vi "update settings and acquire.vi"(8 "error in (no error)":errorcluster, 10 "Settings In":T1, 11 "Queue in":refnum<queue>) -> (0 "error out":errorcluster)   [LabVIEW 2014, in "AvaSpec.lvlib"]
uses:
  AvaSpec.lvlib
  Message Queue/Message Cluster.ctl
  Settings/Settings.ctl
  Acquisition/Hardware Configuration.ctl
  Libraries/AS-5216-DLL/AVS settings.ctl
  Acquisition/Sphere Indicator.ctl
  Settings/Measurement Type.ctl
  Logging/Logging Configuration.ctl
  Message Queue/AvaSpec Message Queue.lvlib
  Acquisition/AvaSpec Acquisition.lvlib
  Logging/AvaSpec Logging.lvlib
  Settings/AvaSpec Settings.lvlib
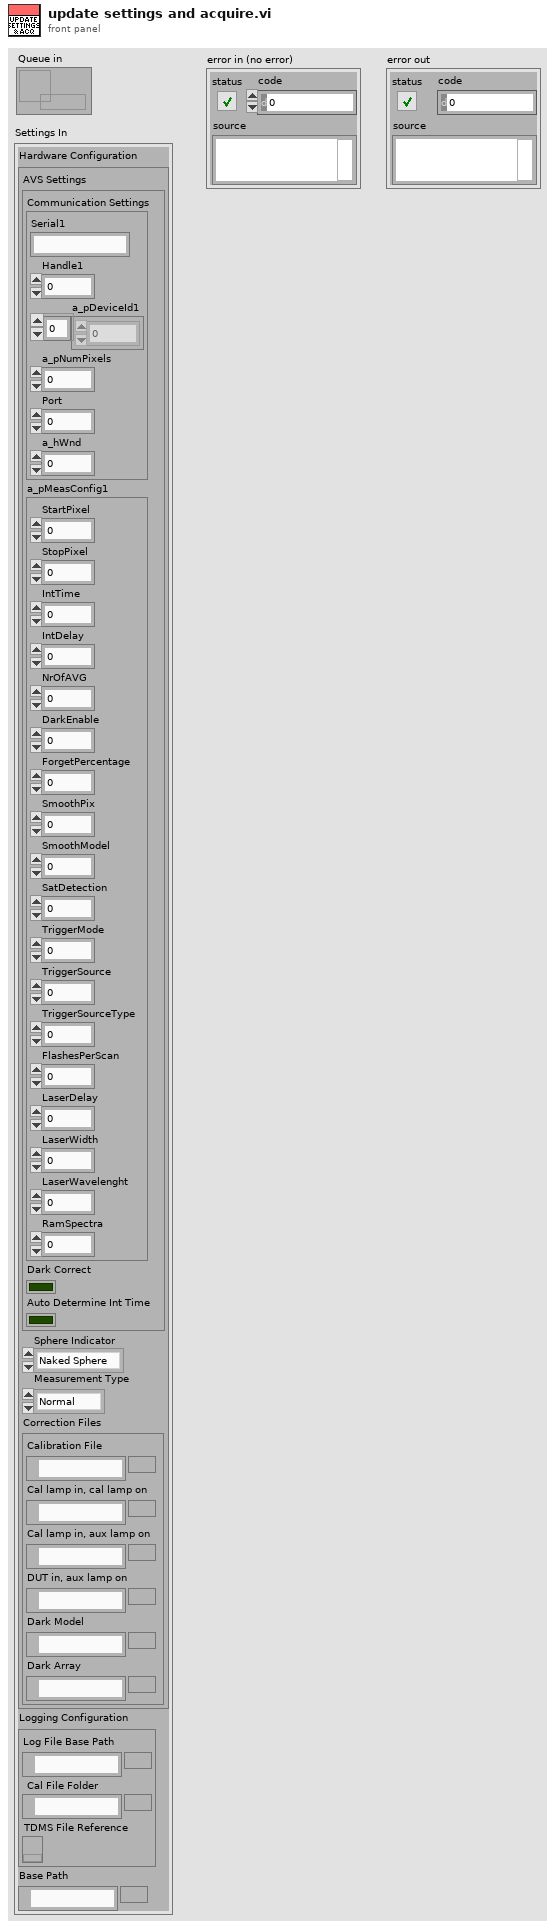
[diagram p1: front panel]
types:
  T1 = typedef "AvaSpec.lvlib/AvaSpec Settings.lvlib/Settings.ctl" = cluster{"Hardware Configuration":T2, "Logging Configuration":T6, "Base Path":path}
  T2 = typedef "AvaSpec.lvlib/AvaSpec Acquisition.lvlib/Hardware Configuration.ctl" = cluster{"AVS Settings":T3, "Sphere Indicator":T4, "Measurement Type":T5, "Correction Files":cluster{"Calibration File":path, "Cal lamp in, cal lamp on":path, "Cal lamp in, aux lamp on":path, "DUT in, aux lamp on":path, "Dark Model":path, "Dark Array":path}}
  T3 = typedef "AvaSpec.lvlib/AVS settings.ctl" = cluster{"Communication Settings":cluster{"Serial1":string, "Handle1":i32, "a_pDeviceId1":u8[], "a_pNumPixels":u16, "Port":i32, "a_hWnd":i32}, "a_pMeasConfig1":cluster{"StartPixel":u16, "StopPixel":u16, "IntTime":sgl, "IntDelay":u32, "NrOfAVG":u32, "DarkEnable":u8, "ForgetPercentage":u8, "SmoothPix":u16, "SmoothModel":u8, "SatDetection":u8, "TriggerMode":u8, "TriggerSource":u8, "TriggerSourceType":u8, "FlashesPerScan":u16, "LaserDelay":u32, "LaserWidth":u32, "LaserWavelenght":sgl, "RamSpectra":u16}, "Dark Correct":bool, "Auto Determine Int Time":bool}
  T4 = typedef "AvaSpec.lvlib/Sphere Indicator.ctl" = enum16{"Naked Sphere", "Insulated Sphere"}
  T5 = typedef "AvaSpec.lvlib/AvaSpec Acquisition.lvlib/Measurement Type.ctl" = enum16{"Normal", "Calibration", "Dark"}
  T6 = typedef "AvaSpec.lvlib/AvaSpec Logging.lvlib/Logging Configuration.ctl" = cluster{"Log File Base Path":path, "Cal File Folder":path, "TDMS File Reference":refnum<k34>}
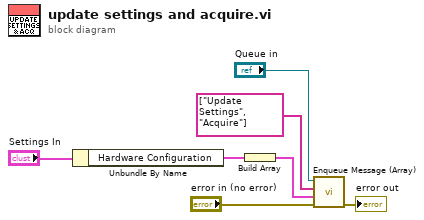
[diagram p0: block diagram]
diagram:
  n1 = Unbundle By Name("Settings In") -> ("Hardware Configuration"=w1:T2)
  n2 = Build Array(w1) -> (w7:T2[])
  n3 = call "Enqueue Message (Array).vi"("error in (no error)"="error in (no error)", "Message Data Array"=w7, "Message Array"=string[] ["Update Settings", "Acquire"], "Message Queue"="Queue in") -> ("error out"=→"error out":errorcluster)  [unwired: 6 in, 1 out]
